vi "Dequeue Message.vi"(8 "error in":errorcluster, 11 "lia host in":refnum<class "LIA Host Interface RT.lvclass">) -> (0 "error out":errorcluster, 1 "timed out?":bool, 2 "message":T1, 3 "lia host out":refnum<class "LIA Host Interface RT.lvclass">)   [LabVIEW 2017, in "LIA Host Interface RT.lvclass"]
uses:
  LIA Host Interface RT.lvclass
  shared/Public/message.ctl
  Properties/IncomingQueue_GET.vi
  shared/Lock-In Amplifier Example Shared.lvlib
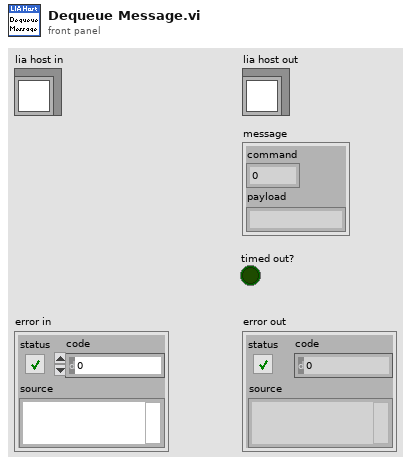
[diagram p1: front panel]
types:
  T1 = typedef "Lock-In Amplifier Example Shared.lvlib/message.ctl" = cluster{"command":u32, "payload":string}
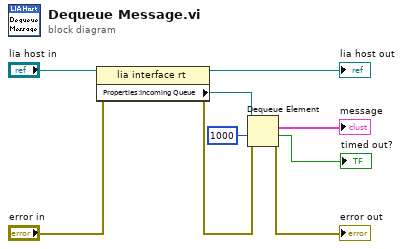
[diagram p0: block diagram]
diagram:
  n1 = property class="lia interface rt"(reference="lia host in", error in="error in") -> (reference out=→"lia host out":refnum<class "LIA Host Interface RT.lvclass">, error out=w7:errorcluster, "Properties:Incoming Queue"=w5:refnum<queue>)
  n2 = Dequeue Element(queue=w5, timeout in ms (-1)=1000, error in (no error)=w7) -> (element=→"message":T1, timed out?=→"timed out?":bool, error out=→"error out":errorcluster)  [unwired: 1 out]
